vi "Get path.vi"(8 "error in (no error)":errorcluster, 11 "system object in":refnum<class "system object.lvclass">) -> (0 "error out":errorcluster, 2 "path":path, 3 "system object out":refnum<class "system object.lvclass">)   [LabVIEW 2020, in "system object.lvclass"]
uses:
  system object.lvclass
  system object.lvclass/system object.ctl
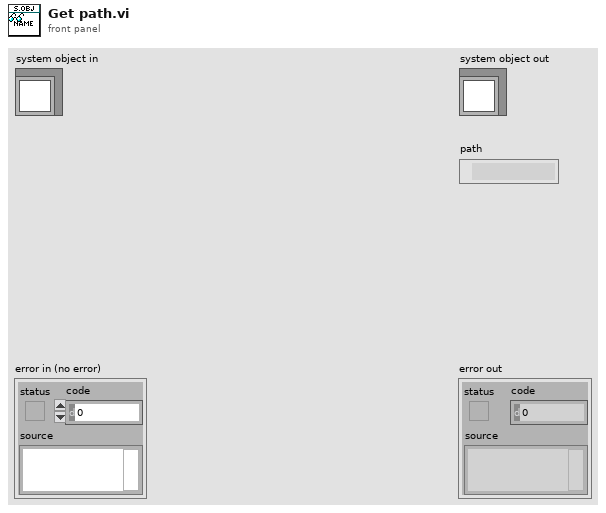
[diagram p1: front panel]
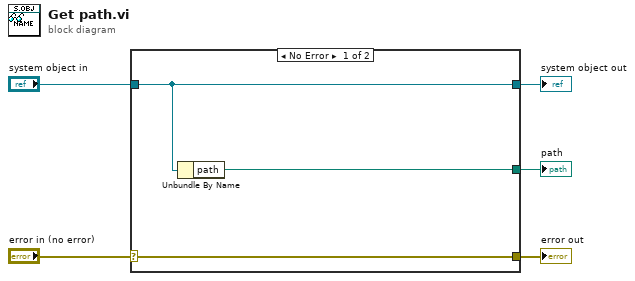
[diagram p0: block diagram]
diagram:
  n1 = case shown="No Error" "error in (no error)" {
    selector: "error in (no error)" -> [w8 w9]
    tunnel: [w8 w9] -> w4
    tunnel: [w7 w10] -> w2
    tunnel: "system object in" -> [w7 w10]
    tunnel: [w6 _] -> w1
    frame No Error {
      n2 = Unbundle By Name(w7) -> ("path"=w6:path)
    }
    frame Error {
    }
  }
  "error out" <- w4
  "system object out" <- w2
  "path" <- w1
